vi "Destroy.vi"   [LabVIEW 2018, in "Toolkit.lvlib" / "Known Host.lvclass"]
uses:
  Known Host.lvclass
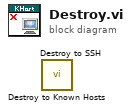
[diagram p0: block diagram]
diagram:
  n1 = call "Destroy to Known Hosts.vi"() -> ()  [unwired: 10 in, 2 out]
  n2 = call "Destroy to SSH.vi"() -> ()  [unwired: 10 in, 2 out]
